vi "niFpgaFFTOutsideSCTLMemWriteLogic.vi"(0 "input data":T2 {"Real" format="%.16g"; "Imaginary" format="%.16g"}, 1 "transfer data":T2 {"Real" format="%.16g"; "Imaginary" format="%.16g"}, 5 "x from bf":T2 {"Real" format="%.16g"; "Imaginary" format="%.16g"}, 7 "y from bf":T2 {"Real" format="%.16g"; "Imaginary" format="%.16g"}, 9 "read address":u16, 12 "control signals":T3) -> (4 "memory output A":T1 {"data"."Real" format="%.16g"; "data"."Imaginary" format="%.16g"}, 6 "memory output B":T1 {"data"."Real" format="%.16g"; "data"."Imaginary" format="%.16g"}, 8 "memory output A 2":T1 {"data"."Real" format="%.16g"; "data"."Imaginary" format="%.16g"}, 10 "memory output B 2":T1 {"data"."Real" format="%.16g"; "data"."Imaginary" format="%.16g"})   [LabVIEW 2017]
uses:
  <vilib>/rvi/Analysis/measure/FFT/templates/niFPGA FFT Outside SCTL Control Signals.ctl
  <vilib>/rvi/FXPMathLib/basic elements/FxpDiscreteDelay/XNode/nifxpmath_DiscreteDelay.xnode
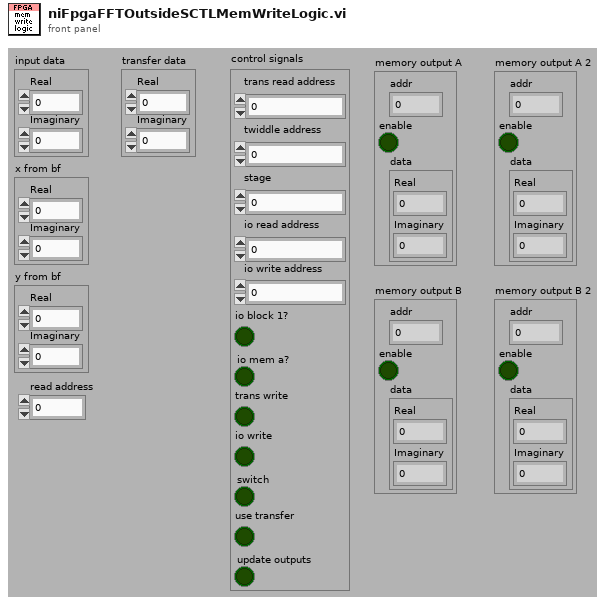
[diagram p1: front panel]
types:
  T1 = cluster{"addr":u16, "enable":bool, "data":cluster{"Real":fxp<+/-,16,1>, "Imaginary":fxp<+/-,16,1>}}
  T2 = cluster{"Real":fxp<+/-,16,1>, "Imaginary":fxp<+/-,16,1>}
  T3 = typedef "niFPGA FFT Outside SCTL Control Signals.ctl" = cluster{"switch":bool, "twiddle address":u16, "stage":u8, "io read address":u16, "io block 1?":bool, "trans write":bool, "io write address":u16, "update outputs":bool, "use transfer":bool, "io mem a?":bool, "io write":bool, "trans read address":u16}
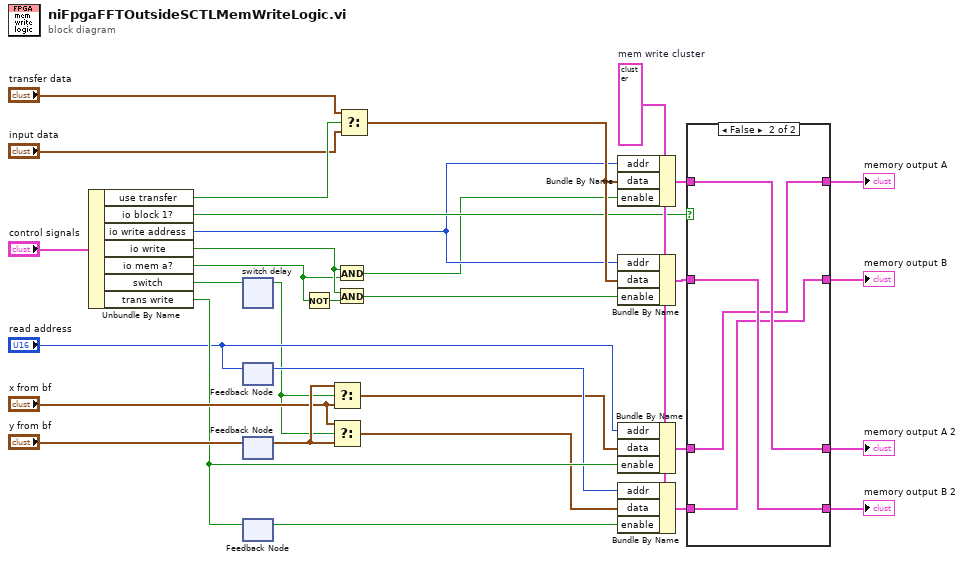
[diagram p0: block diagram]
diagram:
  w24 = T1 {"addr"=0, "enable"=FALSE, "data"={"Real"=0.0, "Imaginary"=0.0}}  # mem write cluster
  n1 = Unbundle By Name("control signals") -> ("use transfer"=w18:bool, "io block 1?"=w17:bool, "io write address"=w16:u16, "io write"=w15:bool, "io mem a?"=w11:bool, "switch"=w10:bool, "trans write"=w27:bool)
  n2 = xnode ("switch delay")("D"=w10) -> ("Q"=w9:bool)
  n3 = feedback-in #1("read address") -> ()
  n4 = feedback #1() -> (w26:u16)  [unwired: 1 out]
  n5 = feedback-in #2("y from bf") -> ()
  n6 = feedback #2() -> (w30:T2)  [unwired: 1 out]
  n7 = feedback-in #3(w27) -> ()
  n8 = feedback #3() -> (w28:bool)  [unwired: 1 out]
  n9 = Not(x=w11) -> (.not. x?=w12:bool)
  n10 = Select(t=w30, s=w9, f="x from bf") -> (s? t:f=w6:T2)
  n11 = Select(t="x from bf", s=w9, f=w30) -> (s? t:f=w5:T2)
  n12 = And(x=w15, y=w11) -> (x .and. y?=w14:bool)
  n13 = And(x=w15, y=w12) -> (x .and. y?=w13:bool)
  n14 = Select(t="transfer data", s=w18, f="input data") -> (s? t:f=w19:T2)
  n15 = Bundle By Name(cluster=w24, "addr"=w16, "data"=w19, "enable"=w14) -> (w22:T1)
  n16 = Bundle By Name(cluster=w24, "addr"=w16, "data"=w19, "enable"=w13) -> (w23:T1)
  n17 = Bundle By Name(cluster=w24, "addr"="read address", "data"=w6, "enable"=w27) -> (w21:T1)
  n18 = Bundle By Name(cluster=w24, "addr"=w26, "data"=w5, "enable"=w28) -> (w20:T1)
  n19 = case shown="False" w17 {
    tunnel: w23 -> [w35 w39]
    tunnel: w22 -> [w36 w40]
    tunnel: w21 -> [w34 w38]
    tunnel: w20 -> [w33 w37]
    tunnel: [w36 w38] -> w4
    tunnel: [w35 w37] -> w3
    tunnel: [w34 w40] -> w2
    tunnel: [w33 w39] -> w1
    frame True {
    }
    frame False {
    }
  }
  "memory output A" <- w4
  "memory output B" <- w3
  "memory output A 2" <- w2
  "memory output B 2" <- w1
